vi "Reset.vi"(0 "VISA resource name":refnum<visa-resource-name>, 1 "Unit Address (1)":u8=1, 11 "error in (no error)":errorcluster {"code" format="%.0x"}) -> (4 "VISA resource name out":refnum<visa-resource-name>, 15 "error out":errorcluster {"code" format="%.0x"})   [LabVIEW 2010]
doc: "This VI resets the instrument, and then sends a set of default setup commands to the instrument. If a Reset command is not supported, it will return a warning."
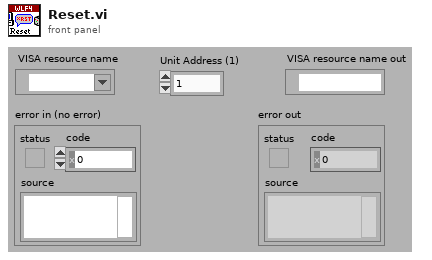
[diagram p1: front panel]
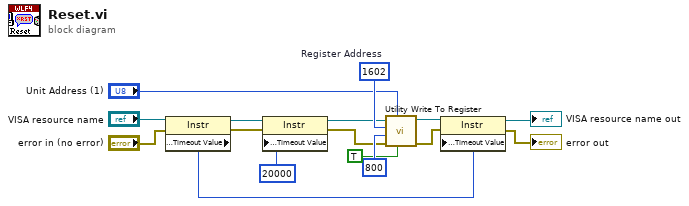
[diagram p0: block diagram]
diagram:
  w16 = u16 1602  # Register Address
  n1 = property class="Instr"(reference="VISA resource name", error in="error in (no error)") -> (reference out=w11:refnum<visa-resource-name>, error out=w4:errorcluster, "General Settings:Timeout Value"=w6:u32)
  n2 = property class="Instr"(reference=w11, error in=w4, "General Settings:Timeout Value"=u32 20000) -> (reference out=w10:refnum<visa-resource-name>, error out=w3:errorcluster)
  n3 = call "Utility Write To Register.vi"("Direct Action?"=TRUE, "Unit Address (1)"="Unit Address (1)", "error in (no error)"=w3, "Data (0)"=i16 800, "Register Address (0)"=w16, "VISA resource name"=w10) -> ("error out"=w2:errorcluster, "VISA resource name out"=w9:refnum<visa-resource-name>)  [unwired: 4 in]
  n4 = property class="Instr"(reference=w9, error in=w2, "General Settings:Timeout Value"=w6) -> (reference out=→"VISA resource name out":refnum<visa-resource-name>, error out=→"error out":errorcluster)
